vi "Show Packages Folder.vi"(8 "Error In":errorcluster, 11 "Target Project Root In":path) -> (0 "Error Out":errorcluster, 3 "Target Project Root Out":path)   [LabVIEW 2017, in "Scripts.lvlib"]
doc: "Newer version of LabVIEW offer the \"Show in File System.vi\", which this VI essentially copies for just the Windows case. The \"Show in File System.vi\" cannot be used because it has a \"Open URL In Browser.vi\" sub-VI for the Linux case that has a password protected block diagram. When this project is saved for a previous version of LabVIEW, a dialog appears asking to verify the password. This can be skipped and everything works fine, but the popup dialog blocks the build and packaging. The user still has to sit and watch the build if the \"Show in File System.vi\" is used."
uses:
  Scripts.lvlib
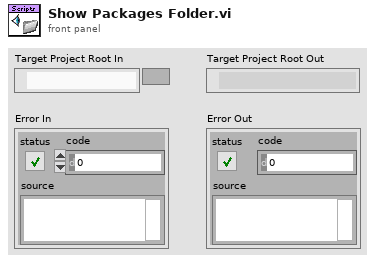
[diagram p1: front panel]
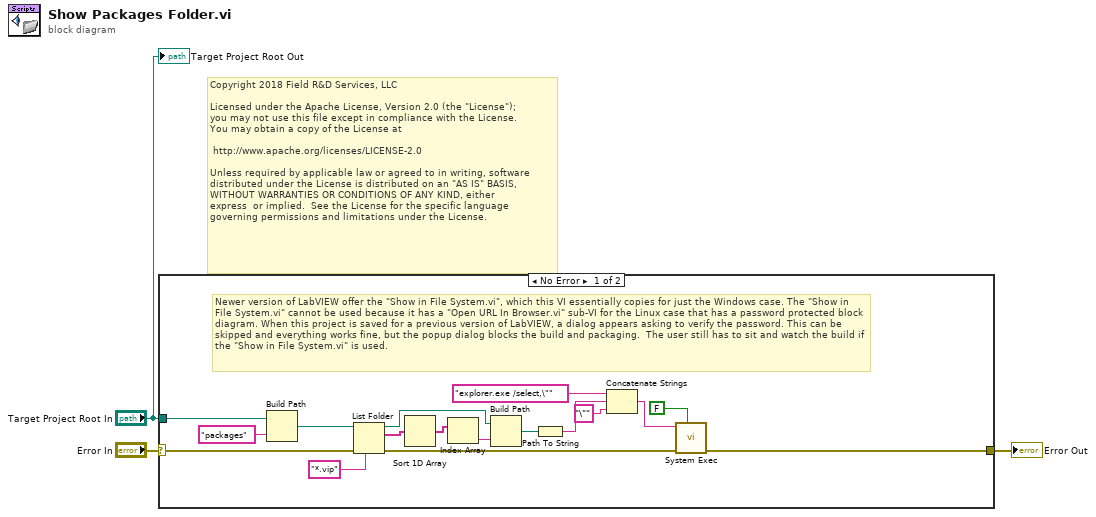
[diagram p0: block diagram]
diagram:
  # "Copyright 2018 Field R&D Services, LLC\n\nLicensed under the Apache License, Version 2.0 (the \"License\");\nyou may not use this file except in compliance with the License.\nYou may obtain a copy of the License at\n\n\thttp://www.apache.org/licenses/LICENSE-2.0\n\nUnless required by applicable law or agreed to in writing, software\ndistributed under the License is distributed on an \"AS IS\" BASIS,\nWITHOUT WARRANTIES OR CONDITIONS OF ANY KIND, either \nexpress  or implied.  See the License for the specific language \ngoverning permissions and limitations under the License."
  n1 = case shown="No Error" "Error In" {
    selector: "Error In" -> [w4 w21]
    tunnel: [w20 w21] -> w3
    tunnel: "Target Project Root In" -> [w18 _]
    frame No Error {
      # "Newer version of LabVIEW offer the \"Show in File System.vi\", which this VI essentially copies for just the Windows case. The \"Show in File System.vi\" cannot be used because it has a \"Open URL In Browser.vi\" sub-VI for the Linux case that has a password protected block diagram. When this project is saved for a previous version of LabVIEW, a dialog appears asking to verify the password. This can be skipped and everything works fine, but the popup dialog blocks the build and packaging.  The user still has to sit and watch the build if the \"Show in File System.vi\" is used."
      n2 = Build Path(base path=w18, name or relative path="packages") -> (appended path=w12:path)
      n3 = List Folder(path=w12, pattern="*.vip", error in=w4) -> (path out=w8:path, filenames=w6:string[], error out=w11:errorcluster)  [unwired: 1 in, 1 out]
      n4 = Sort 1D Array(array=w6) -> (sorted array=w5:string[])
      n5 = Index Array(array=w5) -> (element=w9:string)  [unwired: 1 in]
      n6 = Build Path(base path=w8, name or relative path=w9) -> (appended path=w7:path)
      n7 = Path To String(path=w7) -> (string=w17:string)
      n8 = Concatenate Strings("explorer.exe /select,\"" ("string"), w17, "\"" ("string")) -> (w15:string)
      n9 = call <vilib>:"System Exec.vi"("wait until completion? (T)"=FALSE, "error in (no error)"=w11, "command line"=w15) -> ("error out"=w20:errorcluster)  [unwired: 5 in, 3 out]
    }
    frame Error {
    }
  }
  "Error Out" <- w3
  "Target Project Root Out" <- "Target Project Root In"
